vi "Finish.vi"   [LabVIEW 2019]
doc: "This VI is called just before exiting. It is expected to close I/O refnum, save collected data, etc."
uses:
  <vilib>/Rock Robotics/WPI/Utilities/WPI_GetSetVariantRefNum.vi
types:
  T1 = typedef "WPI_SolenoidDevRef.ctl" = cluster{"DevStatus":errorcluster, "Pneumatics Control Module":u8, "Forward Solenoid Channel":T2, "Reverse Solenoid Channel":T2}
  T2 = typedef "WPI_SolenoidChannel.ctl" = enum8{"Solenoid 0", "Solenoid 1", "Solenoid 2", "Solenoid 3", "Solenoid 4", "Solenoid 5", "Solenoid 6", "Solenoid 7", "Invalid"}
  T3 = typedef "WPI_JoystickDevRef.ctl" = cluster{"Device":T4}
  T4 = typedef "WPI_JoystickDeviceEnum.ctl" = enum16{"USB 0", "USB 1", "USB 2", "USB 3", "USB 4", "USB 5"}
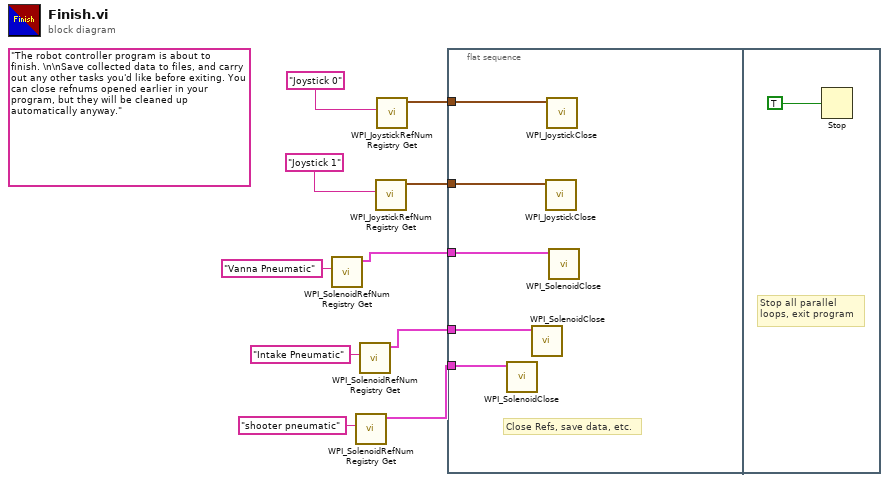
[diagram p0: block diagram]
diagram:
  (unwired) "The robot controller program is about to finish. \n\nSave collected data to files, and carry out any other tasks you'd like before exiting. You can close refnums opened earlier in your program, but they will be cleaned up automatically anyway."
  n1 = call <vilib>:"WPI_SolenoidRefNum Registry Get.vi"("refnum name"="Vanna Pneumatic") -> ("SolenoidDevRef"=w5:T1)  [unwired: 9 in, 1 out]
  n2 = call <vilib>:"WPI_SolenoidRefNum Registry Get.vi"("refnum name"="shooter pneumatic") -> ("SolenoidDevRef"=w1:T1)  [unwired: 9 in, 1 out]
  n3 = call <vilib>:"WPI_SolenoidRefNum Registry Get.vi"("refnum name"="Intake Pneumatic") -> ("SolenoidDevRef"=w3:T1)  [unwired: 9 in, 1 out]
  n4 = call <vilib>:"WPI_JoystickRefNum Registry Get.vi"("refnum name"="Joystick 1") -> ("JoystickDevRef"=w8:T3)  [unwired: 1 in, 9 out]
  n5 = call <vilib>:"WPI_JoystickRefNum Registry Get.vi"("refnum name"="Joystick 0") -> ("JoystickDevRef"=w9:T3)  [unwired: 1 in, 9 out]
  n6 = flat-sequence {
    tunnel: w9 -> [w15]
    tunnel: w8 -> [w14]
    tunnel: w5 -> [w13]
    tunnel: w3 -> [w12]
    tunnel: w1 -> [w11]
    frame #0 {
      # "Close Refs, save data, etc."
      n7 = call <vilib>:"WPI_SolenoidClose.vi"("SolenoidDevRef"=w11) -> ()  [unwired: 10 in, 1 out]
      n8 = call <vilib>:"WPI_SolenoidClose.vi"("SolenoidDevRef"=w12) -> ()  [unwired: 10 in, 1 out]
      n9 = call <vilib>:"WPI_JoystickClose.vi"("JoystickDevRef"=w14) -> ()  [unwired: 11 out]
      n10 = call <vilib>:"WPI_JoystickClose.vi"("JoystickDevRef"=w15) -> ()  [unwired: 11 out]
      n11 = call <vilib>:"WPI_SolenoidClose.vi"("SolenoidDevRef"=w13) -> ()  [unwired: 10 in, 1 out]
    }
    frame #1 {
      # "Stop all parallel\nloops, exit program"
      n12 = Stop(stop? (T)=TRUE ("Quit")) -> ()
    }
  }
